vi "HelloWorldTest.vi"() -> (0 "Array of Error Description":T1)   [LabVIEW 2019]
uses:
  gRPC_ATS/TestUtility/utility.llb/array of error description.ctl
  gRPC_ATS/TestUtility/utility.llb/error description.ctl
  gRPC_ATS/TestUtility/utility.llb/error type.ctl
panel:
  out "Pass":bool
  in  "error in (no error)":errorcluster
  in  "Server VI path":path=path "../../examples/helloworld/helloworld_server/Run greeter_server.vi"
  in  "Client VI Path":path=path "../../examples/helloworld/helloworld_client/Run greeter_client.vi"
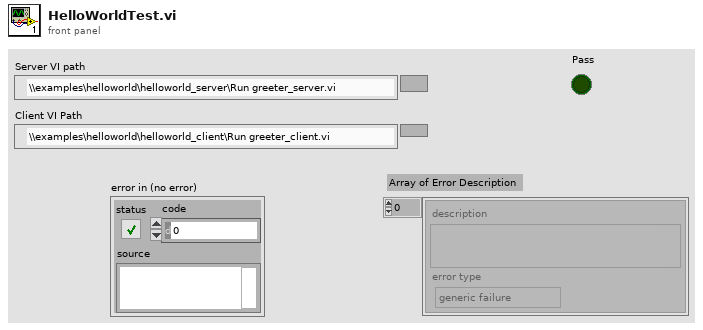
[diagram p1: front panel]
types:
  T1 = typedef "array of error description.ctl" = T2[]
  T2 = typedef "error description.ctl" = cluster{"description":string, "error type":T3}
  T3 = typedef "error type.ctl" = enum32{"generic failure", "boundary case", "precision", "expected error"}
  T4 = typedef "helloworld_client.lvlib/helloworld_HelloReply.ctl" = cluster{"message":string}
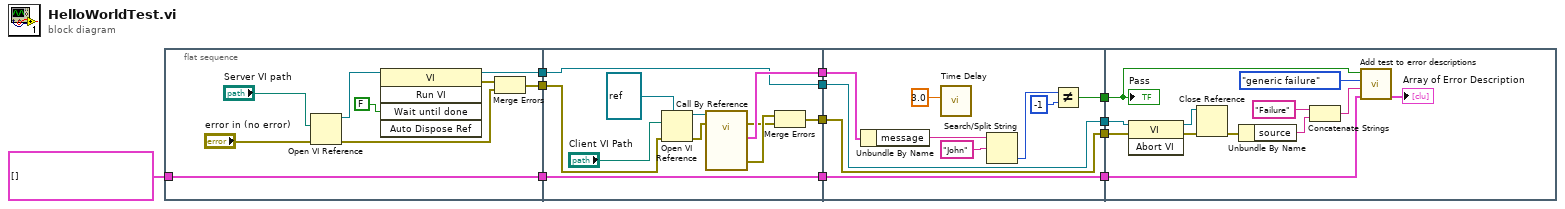
[diagram p0: block diagram]
diagram:
  n1 = flat-sequence {
    tunnel: T1 [] ("error descriptions in") -> [w17]
    tunnel: [w17] -> w9
    tunnel: [w16] -> w2
    tunnel: [w13] -> w1
    tunnel: [w30] -> w12
    tunnel: w9 -> [w31]
    tunnel: [w31] -> w8
    tunnel: [w22] -> w6
    tunnel: [w27] -> w3
    tunnel: w2 -> [w27]
    tunnel: w1 -> [w26]
    tunnel: w12 -> [w40]
    tunnel: [w37] -> w11
    tunnel: w8 -> [w36]
    tunnel: [w36] -> w7
    tunnel: w6 -> [w34]
    tunnel: [w34] -> w5
    tunnel: [w33] -> w4
    tunnel: w3 -> [w33]
    tunnel: w11 -> [w53]
    tunnel: w7 -> [w48]
    tunnel: w5 -> [w43]
    tunnel: w4 -> [w44]
    frame #0 {
      n2 = Open VI Reference(vi path="Server VI path", error in (no error)="error in (no error)") -> (vi reference=w19:refnum<vi>, error out=w15:errorcluster)  [unwired: 4 in]
      n3 = invoke class="VI" method="Run VI"(reference=w19, "Wait until done"=FALSE ("Wait Until Done")) -> (reference out=w16:refnum<vi>, error out=w14:errorcluster)  [unwired: 3 in, 3 out]
      n4 = Merge Errors(w14, w15) -> (w13:errorcluster)
    }
    frame #1 {
      n5 = Open VI Reference(type specifier VI Refnum (for type only)=refnum<vi> refnum, vi path="Client VI Path", error in (no error)=w26) -> (vi reference=w28:refnum<vi>, error out=w25:errorcluster)  [unwired: 3 in]
      n6 = call-by-ref "Call By Reference"(reference=w28, error in=w25) -> (error out=w23:errorcluster, 0:"error out"=w24:errorcluster, "Response Data"=w30:T4)  [unwired: 9 in, 1 out]
      n7 = Merge Errors(w24, w23) -> (w22:errorcluster)
    }
    frame #2 {
      n8 = Unbundle By Name(w40) -> ("message"=w41:string)
      n9 = call "Time Delay"("Delay Time (s)"=3.0) -> ()  [unwired: 10 in, 1 out]
      n10 = Search/Split String(string=w41, search string/char (-)="John") -> (offset of match=w38:i32)  [unwired: 1 in, 2 out]
      n11 = Not Equal?(x=w38, y=-1) -> (x != y?=w37:bool)
    }
    frame #3 {
      n12 = invoke class="VI" method="Abort VI"(reference=w44, error in=w43) -> (reference out=w46:refnum<vi>, error out=w47:errorcluster)  [unwired: 1 in, 1 out]
      n13 = Close Reference(reference=w46, error in (no error)=w47) -> (error out=w45:errorcluster)
      n14 = Unbundle By Name(w45) -> ("source"=w50:string)
      n15 = Concatenate Strings("Failure" ("string"), w50) -> (w51:string)
      n16 = call "Add test to error descriptions.vi"("error descriptions in"=w48, "error string"=w51, "error type"=error_type."generic failure", "pass"=w53) -> ("error description out"=→"Array of Error Description":T1)  [unwired: 3 in]
      "Pass" <- w53
    }
  }
